vi "WriteTravelUnits.vi"(8 "error in":errorcluster, 10 "TravelUnit":T1, 11 "VISA resource name":refnum<visa-resource-name>) -> (0 "error out":errorcluster, 3 "VISA resource name out":refnum<visa-resource-name>)   [LabVIEW 2019, in "Mark 10 TSTM-DC.lvlib"]
uses:
  Mark 10 TSTM-DC.lvlib
  Enum - TravelUnit.ctl
  Mark 10 Event Monitor/Mark 10 Event Monitor.lvlib
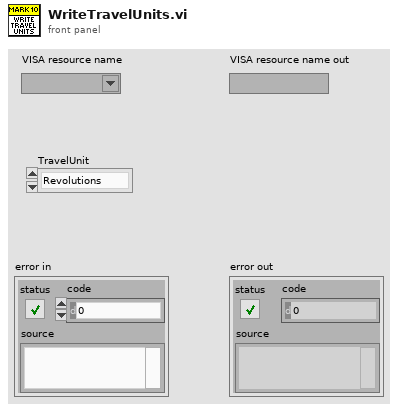
[diagram p1: front panel]
types:
  T1 = typedef "Mark 10 TSTM-DC.lvlib/Enum - TravelUnit.ctl" = enum16{"Revolutions", "Degrees"}
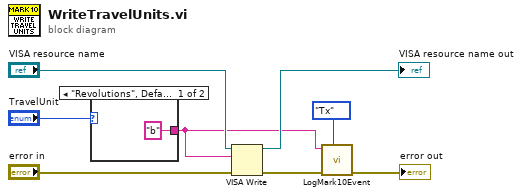
[diagram p0: block diagram]
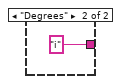
[diagram p2: hidden frame]
diagram:
  n1 = case shown="\"Revolutions\", Default" "TravelUnit" {
    tunnel: ["b" ("String to Write") "i" ("String to Write")] -> w2
    frame "Revolutions", Default {
    }
    frame "Degrees" {
    }
  }
  n2 = VISA Write(VISA resource name="VISA resource name", write buffer=w2, error in (no error)="error in") -> (VISA resource name out=→"VISA resource name out":refnum<visa-resource-name>, error out=w6:errorcluster)  [unwired: 1 out]
  n3 = call "LogMark10Event.vi"("Type"=enum16{"Tx", "Rx"}."Tx", "Error In"=w6, "Event"=w2) -> ("Error Out"=→"error out":errorcluster)  [unwired: 8 in]
